vi "Actor Registry.vi"(6 "Actor Alias":string, 7 "Actor Core Name":string, 8 "Details":T3, 9 "Actor Enqueuer":refnum<class "Message Enqueuer.lvclass">, 10 "Actor ID":string, 11 "Action":T2) -> (0 "All Actors":T1[](array[typedef]), 1 "This Actor":T1, 3 "Found":bool, 4 "Actor Alias out":string, 5 "Event Registration Refnum":refnum<event-registration>)   [LabVIEW 2020, in "Actor Framework.lvlib"]
uses:
  ActorFramework/Message Enqueuer/Message Enqueuer.lvclass
  Registration Mode.ctl
  This Actor.ctl
  ActorFramework/Actor Framework.lvlib
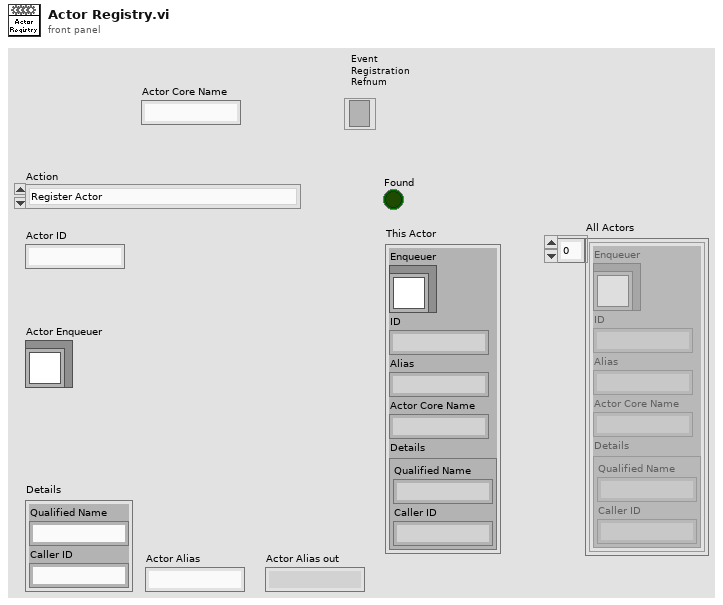
[diagram p1: front panel]
types:
  T1 = typedef "Actor Framework.lvlib/This Actor.ctl" = cluster{"Enqueuer":refnum<class "Message Enqueuer.lvclass">, "ID":string, "Alias":string, "Actor Core Name":string, "Details":cluster{"Qualified Name":string, "Caller ID":string}}
  T2 = typedef "Actor Framework.lvlib/Registration Mode.ctl" = enum16{"Register Actor", "Get ID", "Get Enqueuer", "Deregister Actor", "Get Update Event", "Get All Actors"}
  T3 = cluster{"Qualified Name":string, "Caller ID":string}
  T4 = cluster{"Enqueuers":refnum<class "Message Enqueuer.lvclass">[], "IDs":string[], "Details":cluster{"Qualified Name":string, "Caller ID":string}[], "Aliases":string[], "Cores":string[], "Update Event":refnum<user-event>}
  T5 = cluster{"Qualified Name":string, "Caller ID":string}[]
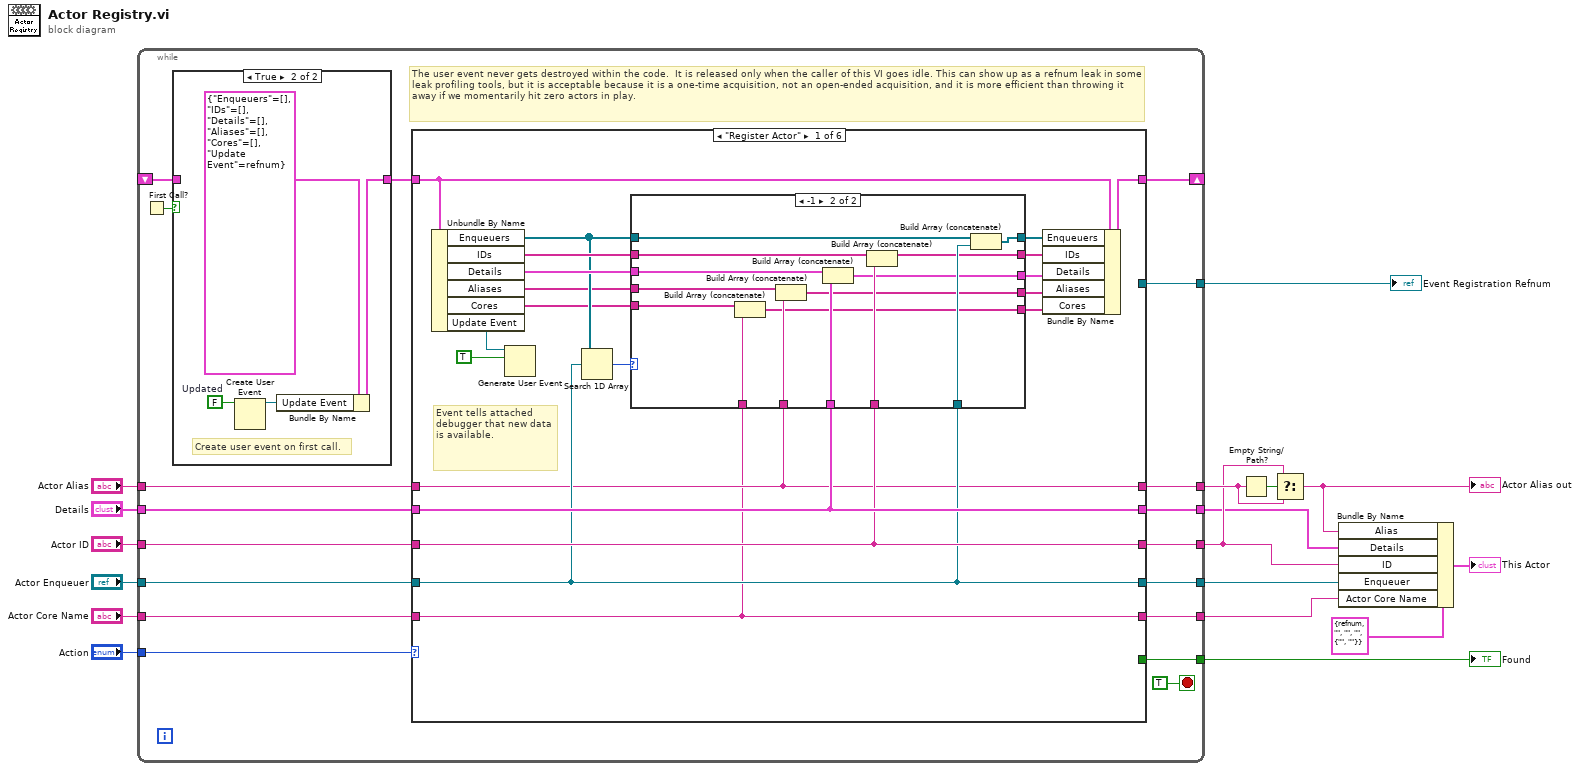
[diagram p0: block diagram]
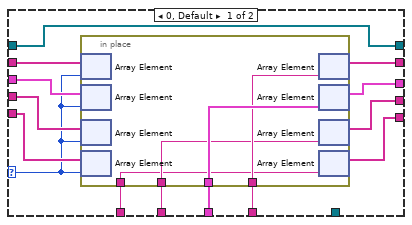
[diagram p3: hidden frame]
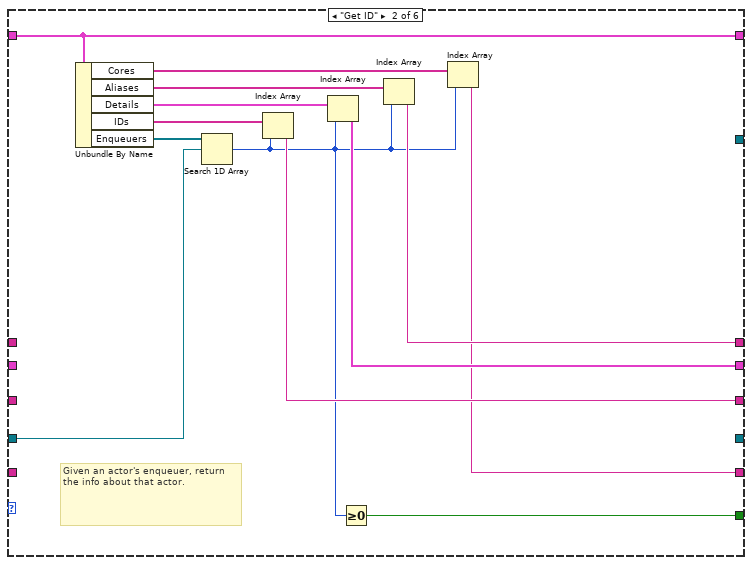
[diagram p4: hidden frame]
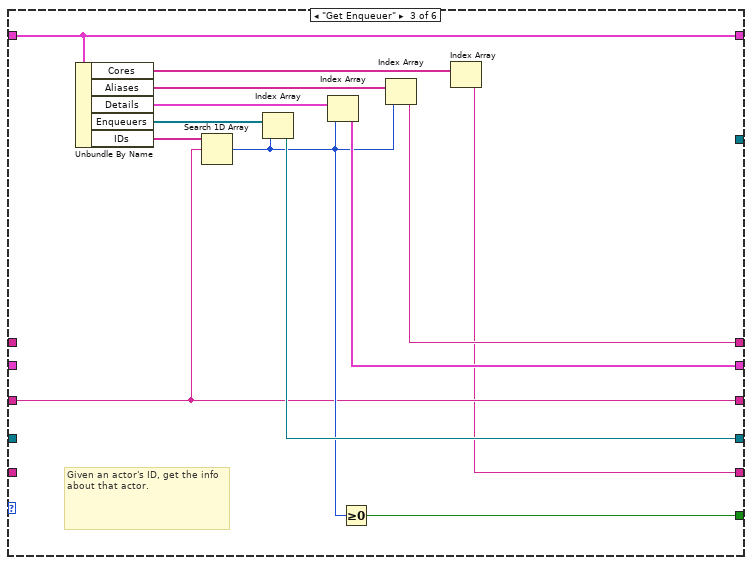
[diagram p5: hidden frame]
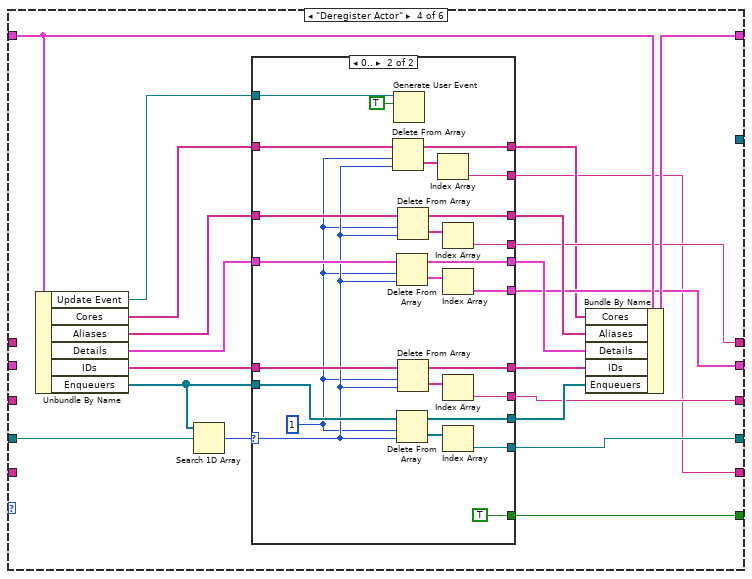
[diagram p6: hidden frame]
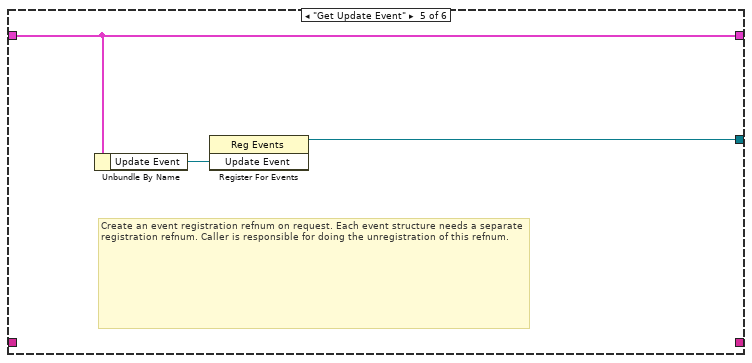
[diagram p8: hidden frame]
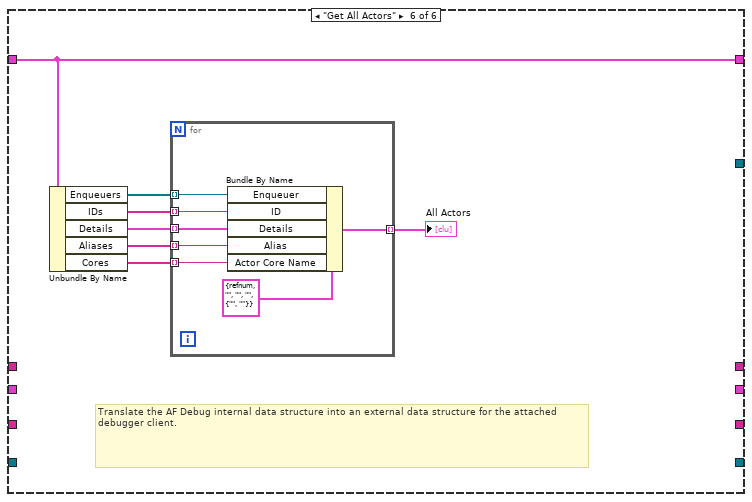
[diagram p9: hidden frame]
diagram:
  n1 = while {
    tunnel: "Action" -> [w35]
    shift-right: [w34] -> _
    shift-left: _ -> [w24]
    tunnel: "Actor ID" -> [w33]
    tunnel: "Actor Enqueuer" -> [w32]
    tunnel: "Details" -> [w31]
    tunnel: [w26] -> w8
    tunnel: [w29] -> w7
    tunnel: [w28] -> w13
    tunnel: [w27] -> w9
    tunnel: "Actor Alias" -> [w22]
    tunnel: [w21] -> w10
    tunnel: "Actor Core Name" -> [w20]
    tunnel: [w19] -> w3
    tunnel: [w18] -> w1
    stop <- TRUE stop-if-true
    # "The user event never gets destroyed within the code.  It is released only when the caller of this VI goes idle. This can show up as a refnum leak in some leak profiling tools, but it is acceptable because it is a one-time acquisition, not an open-ended acquisition, and it is more efficient than throwing it away if we momentarily hit zero actors in play."
    n2 = First Call?() -> (First Call?: T/F=w23:bool)
    n3 = case shown="True" w23 {
      tunnel: [w36 w39] -> w25
      tunnel: w24 -> [w36 _]
      frame False {
      }
      frame True {
        w40 = FALSE  # Updated
        # "Create user event on first call."
        n4 = Create User Event(user event datatype=w40) -> (user event=w38:refnum<user-event>)  [unwired: 1 in, 1 out]
        n5 = Bundle By Name(cluster=T4 {"Enqueuers"=[], "IDs"=[], "Details"=[], "Aliases"=[], "Cores"=[], "Update Event"=refnum}, "Update Event"=w38) -> (w39:T4)
      }
    }
    n6 = case shown="\"Register Actor\"" w35 {
      tunnel: w25 -> [w54 w102 w116 w135 w173 w180]
      tunnel: [w60 w102 w116 w130 w173 w180] -> w34
      tunnel: w33 -> [w48 _ w110 _ _ _]
      tunnel: w32 -> [w47 w105 _ w136 _ _]
      tunnel: w31 -> [w49 _ _ _ _ _]
      tunnel: [w48 w98 w110 w126 _ _] -> w26
      tunnel: [w49 w100 w113 w124 _ _] -> w29
      tunnel: [_ w101 w115 w131 _ _] -> w28
      tunnel: [w47 _ w114 w127 _ _] -> w27
      tunnel: w22 -> [w46 _ _ _ _ _]
      tunnel: [w46 w97 w109 w125 _ _] -> w21
      tunnel: w20 -> [w43 _ _ _ _ _]
      tunnel: [w43 w94 w107 w121 _ _] -> w19
      tunnel: [_ _ _ _ w171 _] -> w18
      frame "Register Actor" {
        # "Event tells attached debugger that new data is available."
        n7 = Unbundle By Name(w54) -> ("Enqueuers"=w53:refnum<class "Message Enqueuer.lvclass">[], "IDs"=w57:string[], "Details"=w56:T5, "Aliases"=w51:string[], "Cores"=w45:string[], "Update Event"=w42:refnum<user-event>)
        n8 = Generate User Event(user event=w42, event data cluster=TRUE ("event data")) -> ()  [unwired: 2 in, 2 out]
        n9 = Search 1D Array(1D array=w53, element=w47) -> (index of element=w52:i32)  [unwired: 1 in]
        n10 = case shown="-1" w52 {
          selector: w52 -> [w63 _]
          tunnel: w48 -> [w72 w93]
          tunnel: w47 -> [_ w92]
          tunnel: w49 -> [w73 w91]
          tunnel: w53 -> [w74 w90]
          tunnel: [w74 w89] -> w59
          tunnel: [w69 w88] -> w58
          tunnel: w57 -> [w71 w87]
          tunnel: w56 -> [w70 w86]
          tunnel: [w68 w85] -> w55
          tunnel: w51 -> [w67 w84]
          tunnel: [w66 w82] -> w50
          tunnel: w46 -> [w65 w83]
          tunnel: w45 -> [w64 w81]
          tunnel: [w62 w80] -> w44
          tunnel: w43 -> [w61 w79]
          frame 0, Default {
            n11 = in-place {
              in-place-border: w73 -> [w78]
              in-place-border: w72 -> [w77]
              in-place-border: w65 -> [w76]
              in-place-border: w61 -> [w75]
              n12 = in-place-array #1(w71, w63) -> ()  [unwired: 1 out]
              n13 = in-place-array #2(w70, w63) -> ()  [unwired: 1 out]
              n14 = in-place-array #3(w67, w63) -> ()  [unwired: 1 out]
              n15 = in-place-array #4(w64, w63) -> ()  [unwired: 1 out]
              n16 = in-place-array #1(w77) -> (w69:string[])  [unwired: 1 out]
              n17 = in-place-array #2(w78) -> (w68:T5)  [unwired: 1 out]
              n18 = in-place-array #3(w76) -> (w66:string[])  [unwired: 1 out]
              n19 = in-place-array #4(w75) -> (w62:string[])  [unwired: 1 out]
            }
          }
          frame -1 {
            n20 = Build Array (concatenate)(w81, w79) -> (w80:string[])
            n21 = Build Array (concatenate)(w84, w83) -> (w82:string[])
            n22 = Build Array (concatenate)(w86, w91) -> (w85:T5)
            n23 = Build Array (concatenate)(w87, w93) -> (w88:string[])
            n24 = Build Array (concatenate)(w90, w92) -> (w89:refnum<class "Message Enqueuer.lvclass">[])
          }
        }
        n25 = Bundle By Name(cluster=w54, "Enqueuers"=w59, "IDs"=w58, "Details"=w55, "Aliases"=w50, "Cores"=w44) -> (w60:T4)
      }
      frame "Get ID" {
        # "Given an actor's enqueuer, return the info about that actor."
        n26 = Unbundle By Name(w102) -> ("Cores"=w96:string[], "Aliases"=w99:string[], "Details"=w104:T5, "IDs"=w103:string[], "Enqueuers"=w106:refnum<class "Message Enqueuer.lvclass">[])
        n27 = Search 1D Array(1D array=w106, element=w105) -> (index of element=w95:i32)  [unwired: 1 in]
        n28 = Index Array(array=w103, index=w95) -> (element=w98:string)
        n29 = Index Array(array=w104, index=w95) -> (element=w100:T3)
        n30 = Greater Or Equal To 0?(x=w95) -> (x >= 0?=w101:bool)
        n31 = Index Array(array=w99, index=w95) -> (element=w97:string)
        n32 = Index Array(array=w96, index=w95) -> (element=w94:string)
      }
      frame "Get Enqueuer" {
        # "Given an actor's ID, get the info about that actor."
        n33 = Unbundle By Name(w116) -> ("Cores"=w108:string[], "Aliases"=w112:string[], "Details"=w118:T5, "Enqueuers"=w117:refnum<class "Message Enqueuer.lvclass">[], "IDs"=w119:string[])
        n34 = Search 1D Array(1D array=w119, element=w110) -> (index of element=w111:i32)  [unwired: 1 in]
        n35 = Index Array(array=w117, index=w111) -> (element=w114:refnum<class "Message Enqueuer.lvclass">)
        n36 = Index Array(array=w118, index=w111) -> (element=w113:T3)
        n37 = Greater Or Equal To 0?(x=w111) -> (x >= 0?=w115:bool)
        n38 = Index Array(array=w112, index=w111) -> (element=w109:string)
        n39 = Index Array(array=w108) -> (element=w107:string)  [unwired: 1 in]
      }
      frame "Deregister Actor" {
        n40 = Unbundle By Name(w135) -> ("Update Event"=w120:refnum<user-event>, "Cores"=w123:string[], "Aliases"=w129:string[], "Details"=w138:T5, "IDs"=w137:string[], "Enqueuers"=w139:refnum<class "Message Enqueuer.lvclass">[])
        n41 = Search 1D Array(1D array=w139, element=w136) -> (index of element=w140:i32)  [unwired: 1 in]
        n42 = case shown="0.." w140 {
          selector: w140 -> [_ w149]
          tunnel: [w144 w170] -> w133
          tunnel: w139 -> [w145 w169]
          tunnel: [w145 w168] -> w134
          tunnel: w137 -> [w144 w167]
          tunnel: [_ TRUE] -> w131
          tunnel: w138 -> [w143 w165]
          tunnel: [w143 w164] -> w132
          tunnel: w129 -> [w142 w163]
          tunnel: [w142 w162] -> w128
          tunnel: [_ w157] -> w127
          tunnel: [_ w156] -> w126
          tunnel: [_ w155] -> w125
          tunnel: [_ w154] -> w124
          tunnel: w123 -> [w141 w152]
          tunnel: [w141 w151] -> w122
          tunnel: [_ w150] -> w121
          tunnel: w120 -> [_ w146]
          frame ..-1 {
          }
          frame 0.. {
            w148 = 1 ("length")
            n43 = Delete From Array(array=w152, length=w148, index=w149) -> (deleted portion=w153:string[], array with subset deleted=w151:string[])
            n44 = Generate User Event(user event=w146, event data cluster=TRUE ("event data")) -> ()  [unwired: 2 in, 2 out]
            n45 = Delete From Array(array=w165, length=w148, index=w149) -> (deleted portion=w160:T5, array with subset deleted=w164:T5)
            n46 = Delete From Array(array=w169, length=w148, index=w149) -> (deleted portion=w158:refnum<class "Message Enqueuer.lvclass">[], array with subset deleted=w168:refnum<class "Message Enqueuer.lvclass">[])
            n47 = Delete From Array(array=w163, length=w148, index=w149) -> (deleted portion=w161:string[], array with subset deleted=w162:string[])
            n48 = Delete From Array(array=w167, length=w148, index=w149) -> (deleted portion=w159:string[], array with subset deleted=w170:string[])
            n49 = Index Array(array=w153) -> (element=w150:string)  [unwired: 1 in]
            n50 = Index Array(array=w161) -> (element=w155:string)  [unwired: 1 in]
            n51 = Index Array(array=w160) -> (element=w154:T3)  [unwired: 1 in]
            n52 = Index Array(array=w159) -> (element=w156:string)  [unwired: 1 in]
            n53 = Index Array(array=w158) -> (element=w157:refnum<class "Message Enqueuer.lvclass">)  [unwired: 1 in]
          }
        }
        n54 = Bundle By Name(cluster=w135, "Cores"=w122, "Aliases"=w128, "Details"=w132, "IDs"=w133, "Enqueuers"=w134) -> (w130:T4)
      }
      frame "Get Update Event" {
        # "Create an event registration refnum on request. Each event structure needs a separate registration refnum. Caller is responsible for doing the unregistration of this refnum."
        n55 = Unbundle By Name(w173) -> ("Update Event"=w172:refnum<user-event>)
        n56 = register-events(w172) -> (reference out=w171:refnum<event-registration>)  [unwired: 2 in, 1 out]
      }
      frame "Get All Actors" {
        # "Translate the AF Debug internal data structure into an external data structure for the attached debugger client."
        n57 = Unbundle By Name(w180) -> ("Enqueuers"=w179:refnum<class "Message Enqueuer.lvclass">[], "IDs"=w178:string[], "Details"=w177:T5, "Aliases"=w176:string[], "Cores"=w175:string[])
        n58 = for {
          tunnel: w179 -> [w186] mode=indexing
          tunnel: w178 -> [w185] mode=indexing
          tunnel: w177 -> [w184] mode=indexing
          tunnel: w176 -> [w183] mode=indexing
          tunnel: w175 -> [w182] mode=indexing
          tunnel: [w181] -> w174 mode=indexing
          n59 = Bundle By Name(cluster=T1 {"Enqueuer"=refnum, "ID"="", "Alias"="", "Actor Core Name"="", "Details"={"Qualified Name"="", "Caller ID"=""}} ("This Actor"), "Enqueuer"=w186, "ID"=w185, "Details"=w184, "Alias"=w183, "Actor Core Name"=w182) -> (w181:T1)
        }
        "All Actors" <- w174
      }
    }
  }
  "Found" <- w13
  "Event Registration Refnum" <- w1
  n60 = Empty String/Path?(string/path=w10) -> (empty?=w11:bool)
  n61 = Select(t=w8, s=w11, f=w10) -> (s? t:f=w6:string)
  "Actor Alias out" <- w6
  n62 = Bundle By Name(cluster=T1 {"Enqueuer"=refnum, "ID"="", "Alias"="", "Actor Core Name"="", "Details"={"Qualified Name"="", "Caller ID"=""}} ("This Actor"), "Alias"=w6, "Details"=w7, "ID"=w8, "Enqueuer"=w9, "Actor Core Name"=w3) -> (→"This Actor":T1)
